vi "CheckoffWaypoint.vi"(8 "Error In":errorcluster, 10 "CurrentLocation":T1 {"North" format="%#_10f"; "East" format="%#_8f"}, 11 "Waypoint In":refnum<class "Waypoint.lvclass">) -> (0 "Error Out":errorcluster, 2 "Done?":bool, 3 "Waypoint Out":refnum<class "Waypoint.lvclass">)   [LabVIEW 2013, in "Waypoint.lvclass"]
doc: "Given a waypoint and the current location, checks whether the waypoint should be checked off, and marks it as done if so."
uses:
  Waypoint.lvclass
  Data/TypeDefs/UTM Location.ctl
  Waypoint.lvclass/Waypoint.ctl
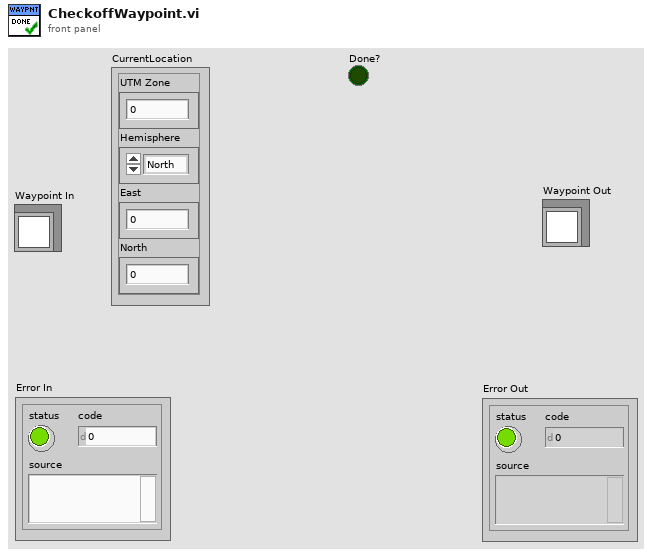
[diagram p1: front panel]
types:
  T1 = typedef "UTM Location.ctl" = cluster{"UTM Zone":dbl, "Hemisphere":enum16{"North", "South"}, "East":dbl, "North":dbl}
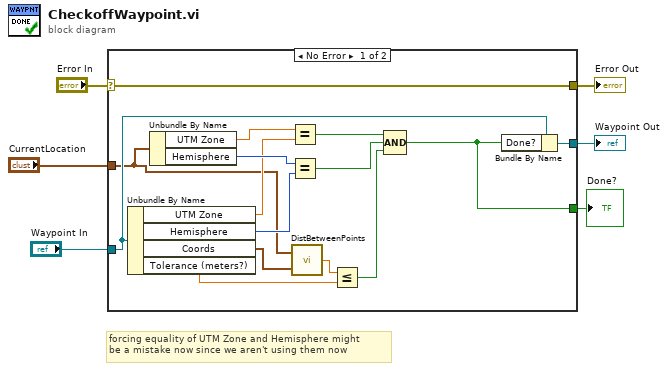
[diagram p0: block diagram]
diagram:
  # "forcing equality of UTM Zone and Hemisphere might\nbe a mistake now since we aren't using them now"
  n1 = case shown="No Error" "Error In" {
    selector: "Error In" -> [w21 w23]
    tunnel: [w21 w23] -> w5
    tunnel: "Waypoint In" -> [w19 w22]
    tunnel: [w20 w22] -> w3
    tunnel: "CurrentLocation" -> [w9 _]
    tunnel: [w7 _] -> w1
    frame No Error {
      n2 = Unbundle By Name(w19) -> ("UTM Zone"=w12:dbl, "Hemisphere"=w13:enum16{"North", "South"}, "Coords"=w10:T1, "Tolerance (meters?)"=w8:dbl)
      n3 = Unbundle By Name(w9) -> ("UTM Zone"=w11:dbl, "Hemisphere"=w14:enum16{"North", "South"})
      n4 = Equal?(x=w11, y=w12) -> (x = y?=w15:bool)
      n5 = Equal?(x=w14, y=w13) -> (x = y?=w16:bool)
      n6 = call "DistBetweenPoints.vi"("UTM Location 2"=w10, "UTM Location"=w9) -> ("Numeric"=w18:dbl)
      n7 = Less Or Equal?(x=w18, y=w8) -> (x <= y?=w17:bool)
      n8 = Compound Arithmetic op=AND(w15, w16, w17) -> (w7:bool)
      n9 = Bundle By Name(cluster=w19, "Done?"=w7) -> (w20:refnum<class "Waypoint.lvclass">)
    }
    frame Error {
    }
  }
  "Waypoint Out" <- w3
  "Error Out" <- w5
  "Done?" <- w1
